vi "Send Command.vi"(8 "error in (no error)":errorcluster, 10 "Command String":string, 11 "Lockin SR830.lvclass In":refnum<class "Lockin SR830.lvclass">) -> (0 "error out":errorcluster, 3 "Lockin SR830.lvclass out":refnum<class "Lockin SR830.lvclass">)   [LabVIEW 2017, in "Lockin SR830.lvclass"]
uses:
  Lockin SR830.lvclass
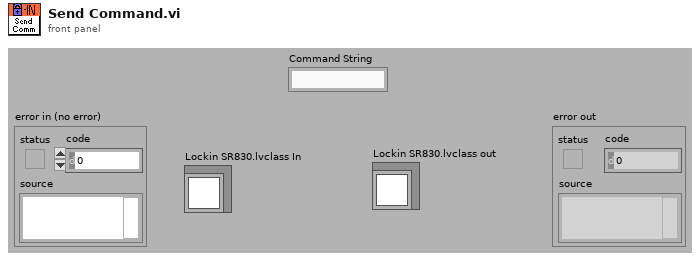
[diagram p1: front panel]
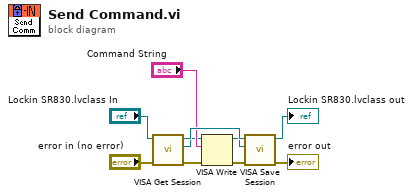
[diagram p0: block diagram]
diagram:
  n1 = call-dynamic "VISA Get Session.vi"("error in (no error)"="error in (no error)", "Instrument.lvclass in"="Lockin SR830.lvclass In") -> ("error out"=w3:errorcluster, "VISA Resource Name"=w4:refnum<visa-resource-name>, "Instrument.lvclass out"=w8:refnum<class "Lockin SR830.lvclass">)  [unwired: 6 in, 1 out]
  n2 = VISA Write(VISA resource name=w4, write buffer="Command String", error in (no error)=w3) -> (VISA resource name out=w2:refnum<visa-resource-name>, error out=w1:errorcluster)  [unwired: 1 out]
  n3 = call-dynamic "VISA Save Session.vi"("error in (no error)"=w1, "VISA Resource Name"=w2, "Instrument.lvclass in"=w8) -> ("error out"=→"error out":errorcluster, "Instrument.lvclass out"=→"Lockin SR830.lvclass out":refnum<class "Lockin SR830.lvclass">)  [unwired: 7 in]
